vi "affine_transform_point.vi"(7 "Inverse Transform":bool, 10 "Pixel Coordinates In":cluster{"X":sgl, "Y":sgl} {"Y" format="%.2f"; "X" format="%.2f"}, 11 "transformation_description":dbl[](array[numeric])) -> (2 "Pixel Coordinates Out":cluster{"X":sgl, "Y":sgl} {"Y" format="%.2f"; "X" format="%.2f"})   [LabVIEW 2019]
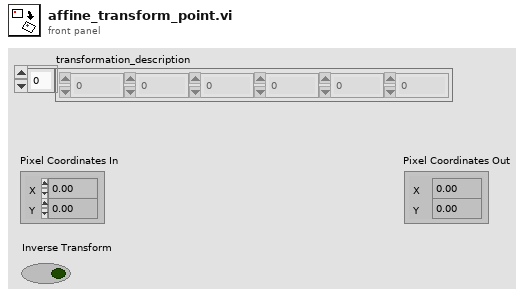
[diagram p1: front panel]
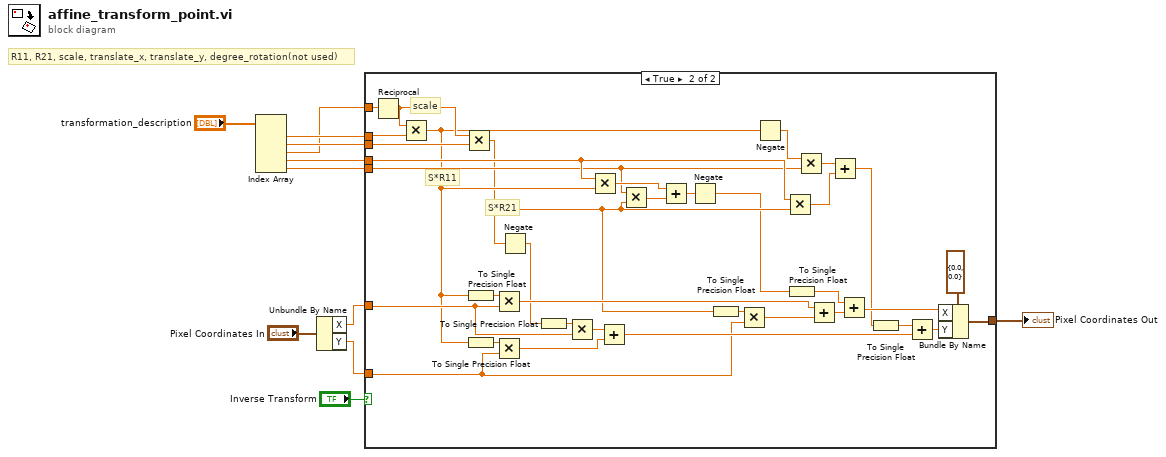
[diagram p0: block diagram]
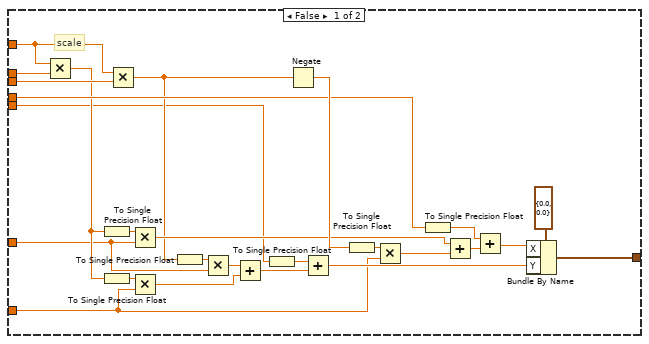
[diagram p2: hidden frame]
diagram:
  # "R11, R21, scale, translate_x, translate_y, degree_rotation(not used)"
  n1 = Index Array(array="transformation_description") -> (element #1=w9:dbl, element #2=w8:dbl, element #3=w5:dbl, element #4=w7:dbl, element #5=w6:dbl)  [unwired: 5 in]
  n2 = Unbundle By Name("Pixel Coordinates In") -> ("X"=w3:sgl, "Y"=w2:sgl)
  n3 = case shown="True" "Inverse Transform" {
    tunnel: w5 -> [w35 w70]
    tunnel: w9 -> [w37 w72]
    tunnel: w8 -> [w36 w71]
    tunnel: w7 -> [w27 w65]
    tunnel: w6 -> [w15 w64]
    tunnel: w3 -> [w18 w44]
    tunnel: w2 -> [w12 w45]
    tunnel: [w13 w38] -> w1
    frame False {
      # "scale"
      n4 = Multiply(x=w35, y=w37) -> (x*y=w23:dbl)
      n5 = To Single Precision Float(number=w23) -> (single precision float=w34:sgl)
      n6 = To Single Precision Float(number=w23) -> (single precision float=w24:sgl)
      n7 = Multiply(x=w35, y=w36) -> (x*y=w21:dbl)
      n8 = Multiply(x=w34, y=w18) -> (x*y=w30:sgl)
      n9 = Multiply(x=w24, y=w12) -> (x*y=w19:sgl)
      n10 = To Single Precision Float(number=w21) -> (single precision float=w22:sgl)
      n11 = Multiply(x=w22, y=w18) -> (x*y=w20:sgl)
      n12 = Add(x=w20, y=w19) -> (x+y=w17:sgl)
      n13 = To Single Precision Float(number=w15) -> (single precision float=w16:sgl)
      n14 = Negate(x=w21) -> (-x=w32:dbl)
      n15 = Add(x=w16, y=w17) -> (x+y=w14:sgl)
      n16 = To Single Precision Float(number=w32) -> (single precision float=w33:sgl)
      n17 = Multiply(x=w33, y=w12) -> (x*y=w31:sgl)
      n18 = To Single Precision Float(number=w27) -> (single precision float=w26:sgl)
      n19 = Add(x=w30, y=w31) -> (x+y=w28:sgl)
      n20 = Add(x=w26, y=w28) -> (x+y=w25:sgl)
      n21 = Bundle By Name(cluster=cluster{"X":sgl, "Y":sgl} {"X"=0.0, "Y"=0.0} ("Pixel Coordinates In"), "X"=w25, "Y"=w14) -> (w13:cluster{"X":sgl, "Y":sgl})
    }
    frame True {
      # "S*R21"
      # "S*R11"
      # "scale"
      n22 = Reciprocal(x=w70) -> (1/x=w69:dbl)
      n23 = Multiply(x=w69, y=w72) -> (x*y=w43:dbl)
      n24 = Multiply(x=w69, y=w71) -> (x*y=w42:dbl)
      n25 = To Single Precision Float(number=w43) -> (single precision float=w60:sgl)
      n26 = To Single Precision Float(number=w43) -> (single precision float=w52:sgl)
      n27 = Multiply(x=w60, y=w44) -> (x*y=w57:sgl)
      n28 = Multiply(x=w52, y=w45) -> (x*y=w49:sgl)
      n29 = Negate(x=w42) -> (-x=w41:dbl)
      n30 = To Single Precision Float(number=w41) -> (single precision float=w51:sgl)
      n31 = Multiply(x=w51, y=w44) -> (x*y=w50:sgl)
      n32 = Multiply(x=w65, y=w43) -> (x*y=w67:dbl)
      n33 = Add(x=w50, y=w49) -> (x+y=w48:sgl)
      n34 = Multiply(x=w64, y=w42) -> (x*y=w68:dbl)
      n35 = Add(x=w67, y=w68) -> (x+y=w66:dbl)
      n36 = Negate(x=w66) -> (-x=w40:dbl)
      n37 = To Single Precision Float(number=w42) -> (single precision float=w59:sgl)
      n38 = Multiply(x=w59, y=w45) -> (x*y=w58:sgl)
      n39 = Negate(x=w43) -> (-x=w63:dbl)
      n40 = Multiply(x=w65, y=w42) -> (x*y=w61:dbl)
      n41 = To Single Precision Float(number=w40) -> (single precision float=w54:sgl)
      n42 = Multiply(x=w63, y=w64) -> (x*y=w62:dbl)
      n43 = Add(x=w57, y=w58) -> (x+y=w55:sgl)
      n44 = Add(x=w62, y=w61) -> (x+y=w39:dbl)
      n45 = Add(x=w54, y=w55) -> (x+y=w53:sgl)
      n46 = To Single Precision Float(number=w39) -> (single precision float=w47:sgl)
      n47 = Add(x=w47, y=w48) -> (x+y=w46:sgl)
      n48 = Bundle By Name(cluster=cluster{"X":sgl, "Y":sgl} {"X"=0.0, "Y"=0.0} ("Pixel Coordinates In"), "X"=w53, "Y"=w46) -> (w38:cluster{"X":sgl, "Y":sgl})
    }
  }
  "Pixel Coordinates Out" <- w1
